vi "SaveFile.vi"(8 "error in (no error)":errorcluster, 11 "VXMCfg in":refnum<class "VXMCfg.lvclass">) -> (0 "error out":errorcluster, 3 "VXMCfg out":refnum<class "VXMCfg.lvclass">)   [LabVIEW 2019, in "VXMCfg.lvclass"]
uses:
  VXMCfg.lvclass
  VXMCfg.ctl
  sub-syst.n.ctl
  VXMCfg.lvclass/VXMCfg.ctl
panel:
  out "VXM Properties":T1
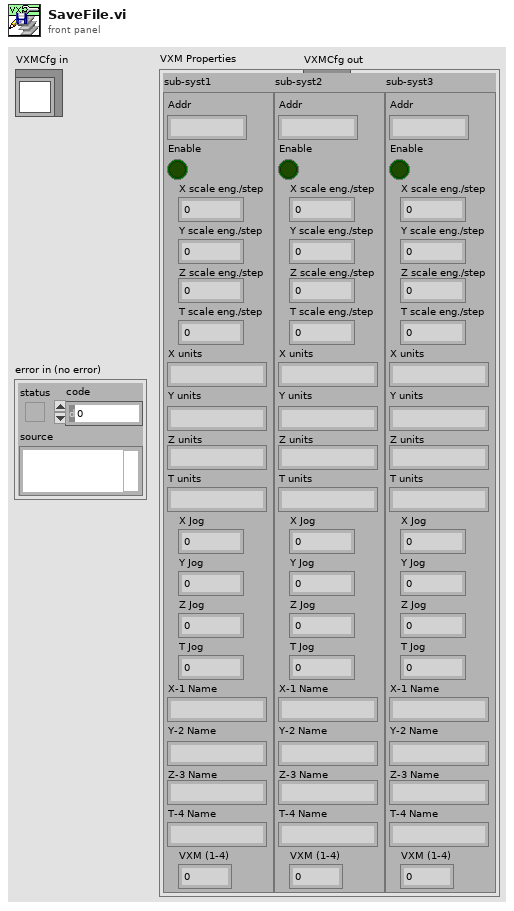
[diagram p1: front panel]
types:
  T1 = typedef "VXMCfg.ctl" = cluster{"sub-syst1":T2, "sub-syst2":T2, "sub-syst3":T2}
  T2 = typedef "sub-syst.n.ctl" = cluster{"Addr":string, "Enable":bool, "X scale eng./step":dbl, "Y scale eng./step":dbl, "Z scale eng./step":dbl, "T scale eng./step":dbl, "X units":string, "Y units":string, "Z units":string, "T units":string, "X Jog":dbl, "Y Jog":dbl, "Z Jog":dbl, "T Jog":dbl, "X-1 Name":string, "Y-2 Name":string, "Z-3 Name":string, "T-4 Name":string, "VXM (1-4)":i32}
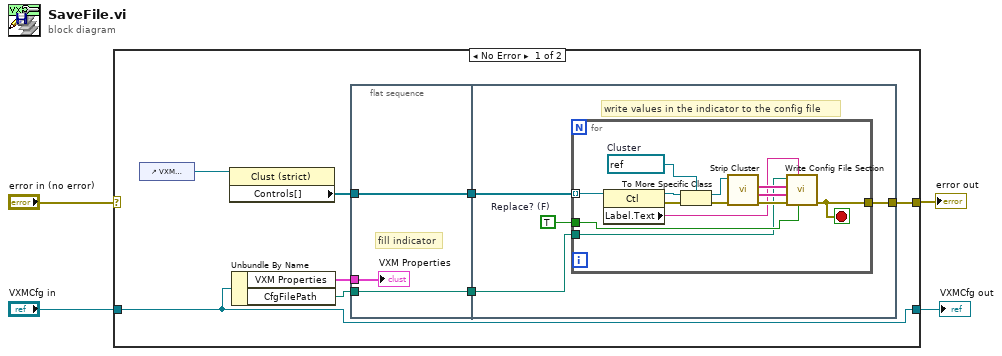
[diagram p0: block diagram]
diagram:
  n1 = case shown="No Error" "error in (no error)" {
    selector: "error in (no error)" -> [_ w34]
    tunnel: [w6 w34] -> w1
    tunnel: [w7 w33] -> w2
    tunnel: "VXMCfg in" -> [w7 w33]
    frame No Error {
      n2 = control-ref of="VXM Properties"() -> (w5:refnum<vi>)
      n3 = property class="Clust (strict)"(reference=w5) -> ("Controls[]"=w10:refnum<vi>[])  [unwired: 1 in, 2 out]
      n4 = Unbundle By Name(w7) -> ("VXM Properties"=w8:T1, "CfgFilePath"=w9:path)
      n5 = flat-sequence {
        tunnel: w8 -> [w13]
        tunnel: w9 -> [w15]
        tunnel: [w15] -> w12
        tunnel: [w14] -> w11
        tunnel: w10 -> [w14]
        tunnel: w12 -> [w16]
        tunnel: w11 -> [w18]
        tunnel: [w17] -> w6
        frame #0 {
          # "fill indicator"
          "VXM Properties" <- w13
        }
        frame #1 {
          w19 = TRUE  # Replace? (F)
          # "write values in the indicator to the config file"
          n6 = for {
            tunnel: [w26] -> w17
            tunnel: w19 -> [w23]
            tunnel: w16 -> [w22]
            tunnel: w18 -> [w21] mode=indexing
            stop <- w26 stop-if-true
            w32 = refnum<vi> refnum  # Cluster
            n7 = property class="Ctl"(reference=w21) -> (reference out=w25:refnum<vi>, error out=w20:errorcluster, "Label.Text"=w24:string)  [unwired: 1 in]
            n8 = To More Specific Class(target class=w32, reference=w25, error in=w20) -> (specific class reference=w31:refnum<vi>, error out=w28:errorcluster)
            n9 = call "Strip Cluster.vi"("error in (no error)"=w28, "Cluster Refnum"=w31) -> ("error out"=w27:errorcluster, "Values"=w29:string[], "Keys"=w30:string[])  [unwired: 6 in, 1 out]
            n10 = call "Write Config File Section.vi"("Replace? (F)"=w23, "Section"=w24, "error in"=w27, "Values"=w29, "Keys"=w30, "INI path"=w22) -> ("error out"=w26:errorcluster)  [unwired: 5 in]
          }
        }
      }
    }
    frame Error {
    }
  }
  "error out" <- w1
  "VXMCfg out" <- w2
